vi "Goto1.vi"(7 "Speed":u32, 8 "error in (no error)":errorcluster, 10 "New Position":u64, 11 "TranslationStage in":refnum<class "KIM101.lvclass">) -> (0 "error out":errorcluster, 3 "TranslationStage out":refnum<class "KIM101.lvclass">)   [LabVIEW 2023, in "KIM101.lvlib" / "KIM101.lvclass"]
uses:
  KIM101.lvclass
  KIM101.lvclass/KIM101.ctl
  C:/Users/quantum/Downloads/SinglePhotonInterferometryUI-master/Thorlabs.MotionControl.KCube.InertialMotorCLI.dll
  Thorlabs.MotionControl.KCube.InertialMotorCLI.dll
  TranslationStagesComm Messages/StageMoveDone Msg/StageMoveDone Msg.lvclass
  <vilib>/ActorFramework/Actor/Actor.lvclass
  C:/Program Files/National Instruments/LabVIEW 2023/vi.lib/ActorFramework/Actor/Actor.lvclass
  C:/Users/quantum/Downloads/SinglePhotonInterferometryUI-master/Libraries/KIM101_Actor/KIM101/KIM101/KIM101.lvclass
  C:/Users/quantum/Downloads/SinglePhotonInterferometryUI-master/Libraries/InitDeinit/InitDeinit.lvclass
  C:/Users/quantum/Downloads/SinglePhotonInterferometryUI-master/Libraries/TranslationStageInterface/TranslationStagesInterface.lvclass
panel:
  in  "channel":i32(ring)=1 items=["Channel1"=1, "Channel2"=2, "Channel3"=3, "Channel4"=4]
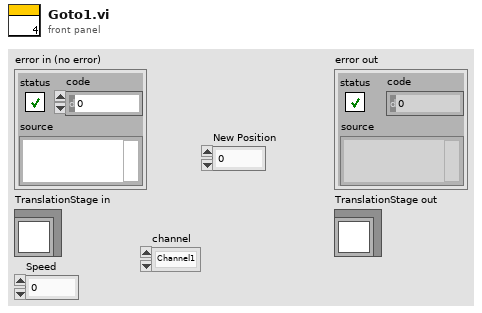
[diagram p1: front panel]
types:
  T1 = cluster{"CH1 Pos":i32, "CH2 Pos":i32, "CH3 Pos":i32, "CH4 Pos":i32}
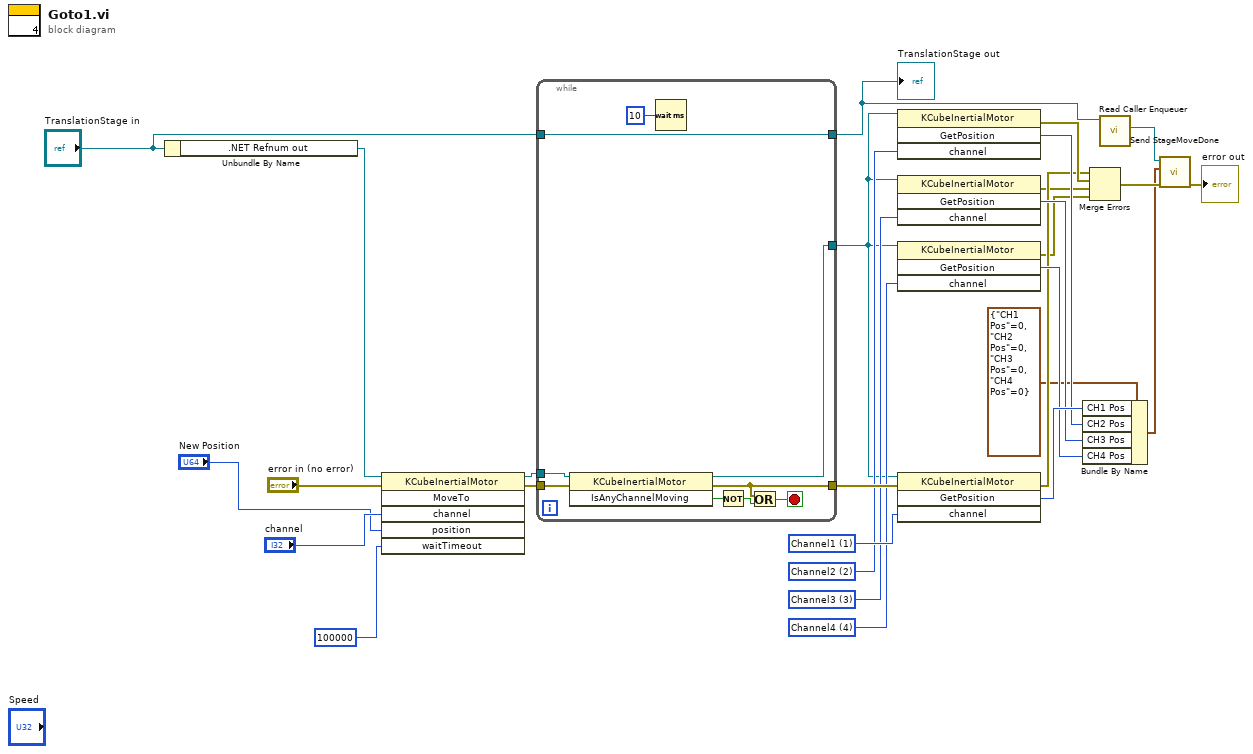
[diagram p0: block diagram]
diagram:
  w14 = 4 items=["Channel1"=1, "Channel2"=2, "Channel3"=3, "Channel4"=4] ("channel")
  w15 = 3 items=["Channel1"=1, "Channel2"=2, "Channel3"=3, "Channel4"=4] ("channel")
  w16 = 2 items=["Channel1"=1, "Channel2"=2, "Channel3"=3, "Channel4"=4] ("channel")
  w17 = 1 items=["Channel1"=1, "Channel2"=2, "Channel3"=3, "Channel4"=4] ("channel")
  n1 = Unbundle By Name("TranslationStage in") -> (".NET Refnum out"=w24:refnum<k24>)
  n2 = invoke class="KCubeInertialMotor" method="MoveTo"(reference=w24, error in="error in (no error)", "channel"="channel", "position"="New Position", "waitTimeout"=100000) -> (reference out=w21:refnum<k24>, error out=w20:errorcluster)  [unwired: 1 in, 4 out]
  n3 = while {
    tunnel: [w34] -> w19
    tunnel: [w37] -> w25
    tunnel: "TranslationStage in" -> [w37]
    tunnel: w21 -> [w32]
    tunnel: w20 -> [w31]
    tunnel: [w29] -> w4
    stop <- w33 stop-if-true
    n4 = invoke class="KCubeInertialMotor" method="IsAnyChannelMoving"(reference=w32, error in=w31) -> (reference out=w29:refnum<k24>, error out=w34:errorcluster, "IsAnyChannelMoving"=w35:bool)  [unwired: 1 in]
    n5 = Wait (ms)(milliseconds to wait=u32 10) -> ()  [unwired: 1 out]
    n6 = Not(x=w35) -> (.not. x?=w30:bool)
    n7 = Or(x=w34, y=w30) -> (x .or. y?=w33:bool)
  }
  "TranslationStage out" <- w25
  n8 = invoke class="KCubeInertialMotor" method="GetPosition"(reference=w4, "channel"=w16) -> (error out=w9:errorcluster, "GetPosition"=w12:i32)  [unwired: 2 in, 2 out]
  n9 = invoke class="KCubeInertialMotor" method="GetPosition"(reference=w4, "channel"=w15) -> (error out=w6:errorcluster, "GetPosition"=w11:i32)  [unwired: 2 in, 2 out]
  n10 = invoke class="KCubeInertialMotor" method="GetPosition"(reference=w4, "channel"=w14) -> (error out=w5:errorcluster, "GetPosition"=w10:i32)  [unwired: 2 in, 2 out]
  n11 = invoke class="KCubeInertialMotor" method="GetPosition"(reference=w4, error in=w19, "channel"=w17) -> (error out=w8:errorcluster, "GetPosition"=w13:i32)  [unwired: 1 in, 2 out]
  n12 = Bundle By Name(cluster=T1 {"CH1 Pos"=0, "CH2 Pos"=0, "CH3 Pos"=0, "CH4 Pos"=0} ("Positions"), "CH1 Pos"=w13, "CH2 Pos"=w12, "CH3 Pos"=w11, "CH4 Pos"=w10) -> (w3:T1)
  n13 = Merge Errors(w8, w9, w6, w5) -> (w7:errorcluster)
  n14 = call <vilib>:"Read Caller Enqueuer.vi"("Actor"=w25) -> ("Caller Enqueuer"=w27:refnum<class "Message Enqueuer.lvclass">)  [unwired: 10 in]
  n15 = call "Send StageMoveDone.vi"("error in (no error)"=w7, "output cluster"=w3, "Message Enqueuer"=w27) -> ("error out"=→"error out":errorcluster)  [unwired: 7 in, 1 out]
